vi "Actor Core.vi"(8 "error in":errorcluster, 11 "Settings Actor in":refnum<class "Settings Actor.lvclass">) -> (0 "error out":errorcluster, 3 "Actor out":refnum<class "Actor.lvclass">)   [LabVIEW 2021, in "Settings Module.lvlib" / "Settings Actor.lvclass"]
doc: "The user interface for this panel.\n\n----\nPlease see the following web address for additional documentation and tutorial information:\nhttp://www.mooregoodideas.com/mgi-panel-manager/\n\nAuthor: Derek Trepanier\n\nCopyright (c) 2018, Moore Good Ideas, Inc.\n\nAll rights reserved.\n\nRedistribution and use in source and binary forms, with or without modification, are permitted provided that the following conditions are met:\n\n * Redistributions of source code must retain the above copyright notice, this list of conditions and the following disclaimer.\n * Redistributions in binary form must reproduce the above copyright notice, this list of conditions and the following disclaimer in the documentation and/or other materials provided with the distribution.\n * Neither the name of Moore Good Ideas, Inc. nor the names of its contributors may be used to endorse or promote products derived from this software without specific prior written permission.\n\nTHIS SOFTWARE IS PROVIDED BY THE COPYRIGHT HOLDERS AND CONTRIBUTORS \"AS IS\" AND ANY EXPRESS OR IMPLIED WARRANTIES, INCLUDING, BUT NOT LIMITED TO, THE IMPLIED WARRANTIES OF MERCHANTABILITY AND FITNESS FOR A PARTICULAR PURPOSE ARE DISCLAIMED. IN NO EVENT SHALL THE COPYRIGHT OWNER OR CONTRIBUTORS BE LIABLE FOR ANY DIRECT, INDIRECT, INCIDENTAL, SPECIAL, EXEMPLARY, OR CONSEQUENTIAL DAMAGES (INCLUDING, BUT NOT LIMITED TO, PROCUREMENT OF SUBSTITUTE GOODS OR SERVICES; LOSS OF USE, DATA, OR PROFITS; OR BUSINESS INTERRUPTION) HOWEVER CAUSED AND ON ANY THEORY OF LIABILITY, WHETHER IN CONTRACT, STRICT LIABILITY, OR TORT (INCLUDING NEGLIGENCE OR OTHERWISE) ARISING IN ANY WAY OUT OF THE USE OF THIS SOFTWARE, EVEN IF ADVISED OF THE POSSIBILITY OF SUCH DAMAGE."
uses:
  Settings Actor.lvclass
  C:/Program Files (x86)/National Instruments/LabVIEW 2021/vi.lib/MGI/Panel Manager/Panel Actor/Panel Actor/Panel Actor.lvclass
  <vilib>/ActorFramework/Actor/Actor.lvclass
  <vilib>/ActorFramework/Message Enqueuer/Message Enqueuer.lvclass/Message Enqueuer.ctl
  <vilib>/ActorFramework/Message Enqueuer/Enqueue.vi
  <vilib>/ActorFramework/Stop Msg/Stop Msg.lvclass
  C:/Program Files (x86)/National Instruments/LabVIEW 2021/vi.lib/ActorFramework/Message/Message.lvclass
  Appearance Actor/Appearance Actor Messages/UI Event-Title Bar-Mouse Down Msg/UI Event-Title Bar-Mouse Down Msg.lvclass
  Appearance Actor/Appearance Actor Messages/UI Event-Close-Value Change Msg/UI Event-Close-Value Change Msg.lvclass
  Appearance Actor/Appearance Actor Messages/UI Event-Maximize-Value Change Msg/UI Event-Maximize-Value Change Msg.lvclass
  Appearance Actor/Appearance Actor Messages/UI Event-Minimize-Value Change Msg/UI Event-Minimize-Value Change Msg.lvclass
  Appearance Actor/Appearance Actor Messages/UI Event-Undock-Value Change Msg/UI Event-Undock-Value Change Msg.lvclass
  <vilib>/ActorFramework/Message Priority Queue/Priority Enqueue.vi
  Appearance Actor/Appearance Actor/Appearance Actor.lvclass
  <vilib>/MGI/Panel Manager/Panel Actor/Panel Actor/Panel Actor.lvclass
  <vilib>/MGI/Panel Manager/Panel Actor/Panel Actor Messages/Show Panel Msg/Show Panel Msg.lvclass
panel:
  in  "Title Bar L":bool
  out "TB.Icon":u16(ring)
  in  "Title Bar M":bool
  out "TB.Title":string
  in  "TB.Light-Button.Undock":bool
  in  "TB.Light-CloseButton":bool
  in  "TB.Light-Button.Maximize":bool
  in  "TB.Light-Button.Minimize":bool
  in  "TB.Dark-Button.Undock":bool
  in  "TB.Dark-CloseButton":bool
  in  "TB.Dark-Button.Maximize":bool
  in  "TB.Dark-Button.Minimize":bool
  in  "Title Bar R":bool
  in  "SM.Light-RadioButton":T1(radio) caption="Radio Buttons"
  in  "SM.Dark-RadioButton":T1(radio) caption="Radio Buttons"
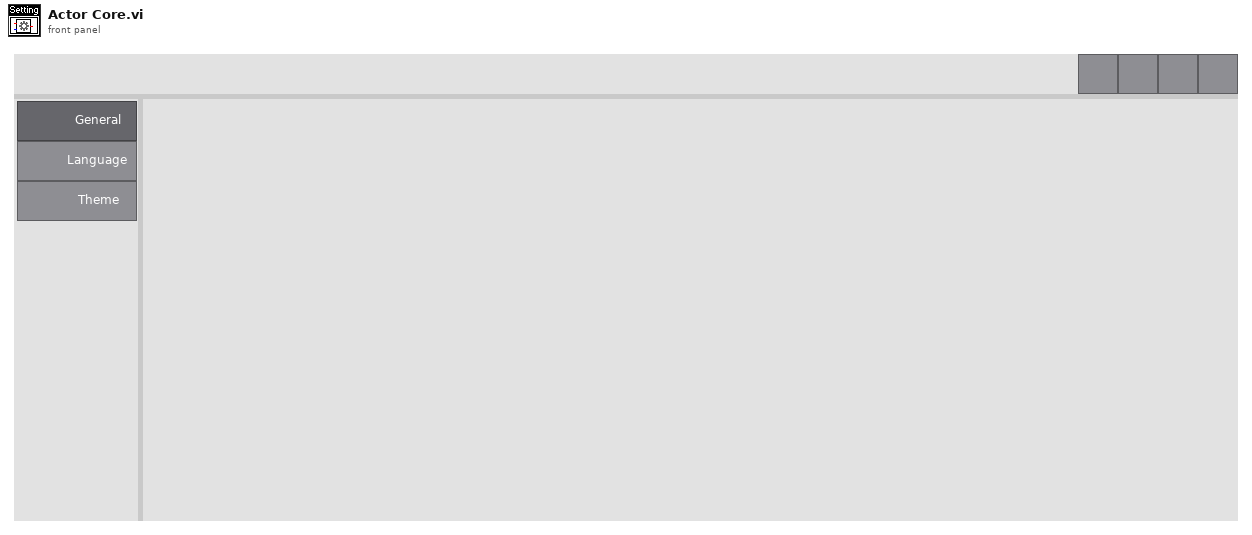
[diagram p1: front panel]
types:
  T1 = enum32{"SM.RadioButton.General", "SM.RadioButton.Language", "SM.RadioButton.Theme"}
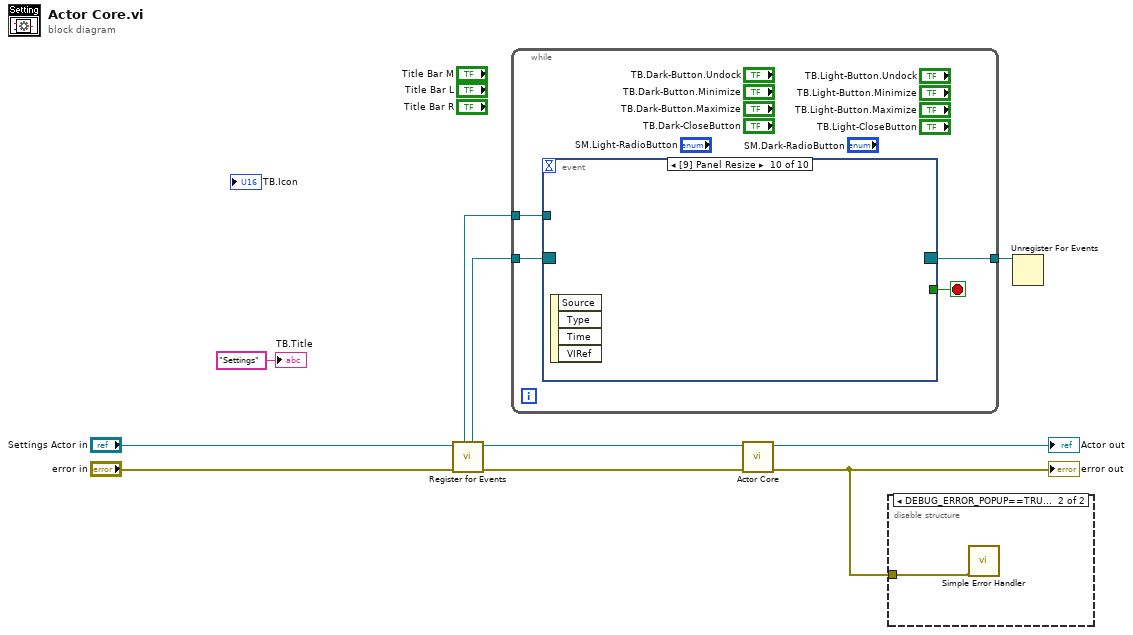
[diagram p0: block diagram]
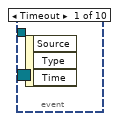
[diagram p3: hidden frame]
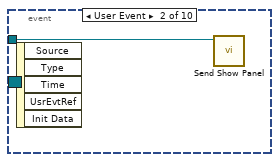
[diagram p4: hidden frame]
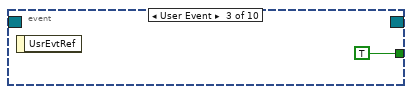
[diagram p5: hidden frame]
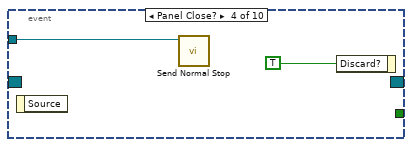
[diagram p6: hidden frame]
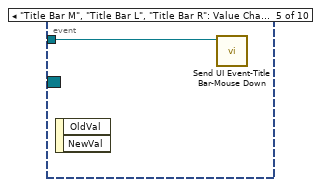
[diagram p7: hidden frame]
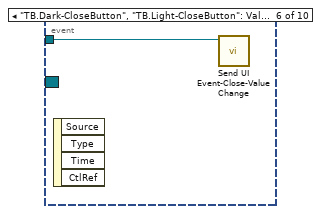
[diagram p8: hidden frame]
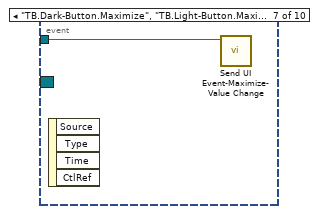
[diagram p9: hidden frame]
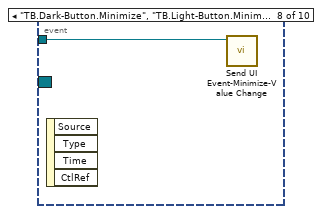
[diagram p10: hidden frame]
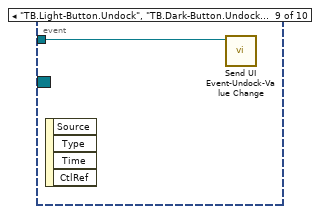
[diagram p11: hidden frame]
diagram:
  n1 = call <vilib>:"Register for Events.vi"("Error In"="error in", "Panel Actor in"="Settings Actor in") -> ("Error Out"=w6:errorcluster, "Panel Actor out"=w4:refnum<class "Settings Actor.lvclass">, "Pnl Actor"=w2:refnum<event-registration>, "Self Enqueuer"=w3:refnum<class "Message Enqueuer.lvclass">)  [unwired: 6 in]
  n2 = while {
    tunnel: w2 -> [w14]
    tunnel: w3 -> [w13]
    tunnel: [w11] -> w7
    stop <- w12 stop-if-true
    n3 = event shown="[9] Panel Resize" {
      selector: w14 -> [_ _ _ _ _ _ _ _ _ _]
      dyn-events: [_ _ _ _ _ _ _ _ _ _] -> w11
      timeout: _ -> [_ _ _ _ _ _ _ _ _ _]
      tunnel: w13 -> [_ w15 _ w18 w19 w20 w21 w22 w23 _]
      tunnel: [_ _ TRUE _ _ _ _ _ _ _] -> w12
      event Timeout {
        n4 = event-data() -> ()  [unwired: 1 in, 3 out]
      }
      event User Event {
        n5 = event-data() -> ()  [unwired: 1 in, 5 out]
        n6 = call <vilib>:"Send Show Panel.vi"("Message Enqueuer in"=w15) -> ()  [unwired: 9 in, 2 out]
      }
      event User Event {
        n7 = event-data() -> ()  [unwired: 1 in, 1 out]
      }
      event Panel Close? {
        n8 = event-data() -> ()  [unwired: 1 in, 1 out]
        n9 = call <vilib>:"Send Normal Stop.vi"("Message Enqueuer"=w18) -> ()  [unwired: 10 in, 1 out]
        n10 = event-data("Discard?"=TRUE) -> ()  [unwired: 1 in, 1 out]
      }
      event "Title Bar M", "Title Bar L", "Title Bar R": Value Change {
        n11 = event-data() -> ()  [unwired: 1 in, 2 out]
        n12 = call "Send UI Event-Title Bar-Mouse Down.vi"("Message Enqueuer"=w19) -> ()  [unwired: 9 in, 2 out]
      }
      event "TB.Dark-CloseButton", "TB.Light-CloseButton": Value Change {
        n13 = event-data() -> ()  [unwired: 1 in, 4 out]
        n14 = call "Send UI Event-Close-Value Change.vi"("Message Enqueuer"=w20) -> ()  [unwired: 9 in, 2 out]
      }
      event "TB.Dark-Button.Maximize", "TB.Light-Button.Maximize": Value Change {
        n15 = event-data() -> ()  [unwired: 1 in, 4 out]
        n16 = call "Send UI Event-Maximize-Value Change.vi"("Message Enqueuer"=w21) -> ()  [unwired: 9 in, 2 out]
      }
      event "TB.Dark-Button.Minimize", "TB.Light-Button.Minimize": Value Change {
        n17 = event-data() -> ()  [unwired: 1 in, 4 out]
        n18 = call "Send UI Event-Minimize-Value Change.vi"("Message Enqueuer"=w22) -> ()  [unwired: 9 in, 2 out]
      }
      event "TB.Light-Button.Undock", "TB.Dark-Button.Undock": Value Change {
        n19 = event-data() -> ()  [unwired: 1 in, 4 out]
        n20 = call "Send UI Event-Undock-Value Change.vi"("Message Enqueuer"=w23) -> ()  [unwired: 9 in, 2 out]
      }
      event Panel Resize {
        n21 = event-data() -> ()  [unwired: 1 in, 4 out]
      }
    }
  }
  n22 = call-parent "Actor Core.vi"("error in"=w6, "Appearance Actor in"=w4) -> ("error out"=w1:errorcluster, "Actor out"=→"Actor out":refnum<class "Actor.lvclass">)  [unwired: 8 in]
  "error out" <- w1
  n23 = disable-structure shown="DEBUG_ERROR_POPUP==TRUE" {
    disable-tunnel: w1 -> [_ w24]
    frame condition #0 {
    }
    frame condition #1 (active) {
      n24 = call <vilib>:"Simple Error Handler.vi"("error in (no error)"=w24) -> ()  [unwired: 4 in, 5 out]
    }
  }
  n25 = Unregister For Events(event registration refnum=w7) -> ()  [unwired: 1 in, 1 out]
  "TB.Title" <- "Settings" ("TB.Title")
